vi "Section File Save.vi"(8 "error in (no error)":errorcluster, 10 "Section File Path":path, 11 "Section Reference in":u64 format="%.0x") -> (0 "error out":errorcluster, 3 "Section Reference out":u64 format="%.0x")   [LabVIEW 2013, in "Hierarchy Framework.lvlib" / "Section.lvclass"]
doc: "Save current section data as a binary file."
uses:
  Section.lvclass
  Generic/Generic.lvclass
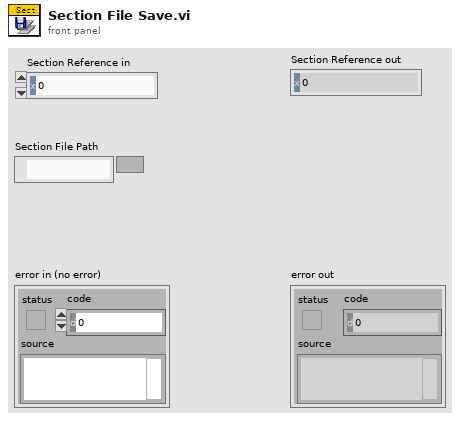
[diagram p1: front panel]
types:
  T1 = enum16{"open", "replace", "create", "open or create", "replace or create", "replace or create with confirmation"}
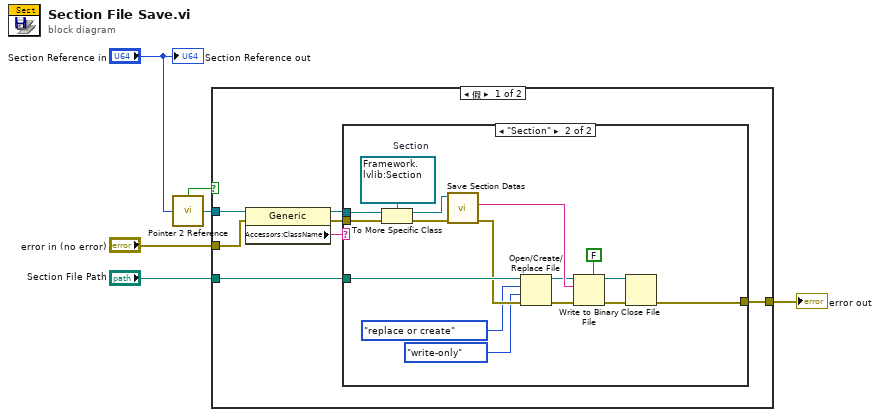
[diagram p0: block diagram]
diagram:
  n1 = call "Pointer 2 Reference.vi"("Pointer"="Section Reference in") -> ("Not A Refnum?"=w5:bool, "Generic Reference"=w4:refnum<data-value>)
  n2 = case shown="假" w5 {
    tunnel: w4 -> [w10 _]
    tunnel: "error in (no error)" -> [w9 w31]
    tunnel: [w8 w31] -> w2
    tunnel: "Section File Path" -> [w7 _]
    frame False {
      n3 = property class="Generic"(reference=w10, error in=w9) -> (reference out=w12:refnum<data-value>, error out=w13:errorcluster, "Accessors:ClassName"=w11:string)
      n4 = case shown="\"Section\"" w11 {
        tunnel: [w14 w25] -> w8
        tunnel: w13 -> [w14 w29]
        tunnel: w12 -> [_ w28]
        tunnel: w7 -> [_ w24]
        frame Default {
        }
        frame "Section" {
          w30 = refnum<data-value> refnum  # Section
          n5 = To More Specific Class(target class=w30, reference=w28, error in=w29) -> (specific class reference=w27:refnum<data-value>, error out=w26:errorcluster)
          n6 = call "Save Section Datas.vi"("error in (no error)"=w26, "Section in"=w27) -> ("error out"=w22:errorcluster, "Data"=w23:string)  [unwired: 7 in, 1 out]
          n7 = Open/Create/Replace File(file path (use dialog)=w24, error in=w22, operation (0:open)=T1."replace or create" ("操作(0:open)"), access (0:read/write)=enum16{"read/write", "read-only", "write-only"}."write-only" ("权限(0:read/write)")) -> (refnum out=w20:refnum<file>, error out=w21:errorcluster)  [unwired: 2 in, 1 out]
          n8 = Write to Binary File(file (use dialog)=w20, data=w23, error in=w21, 5:FALSE ("预置数组或字符串大小？(T)")) -> (refnum out=w17:refnum<file>, error out=w18:errorcluster)  [unwired: 2 in, 1 out]
          n9 = Close File(refnum=w17, error in=w18) -> (error out=w25:errorcluster)  [unwired: 1 out]
        }
      }
    }
    frame True {
    }
  }
  "error out" <- w2
  "Section Reference out" <- "Section Reference in"
